vi "Climb elevator gearing.vi"(11 "Input RPM":dbl) -> (3 "Output RPM":dbl)   [LabVIEW 2019]
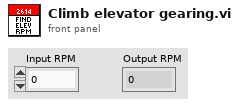
[diagram p1: front panel]
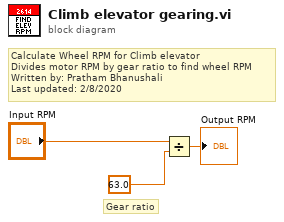
[diagram p0: block diagram]
diagram:
  # "Gear ratio"
  # "Calculate Wheel RPM for Climb elevator\nDivides motor RPM by gear ratio to find wheel RPM\nWritten by: Pratham Bhanushali\nLast updated: 2/8/2020"
  n1 = Divide(x="Input RPM", y=63.0) -> (x/y=→"Output RPM":dbl)
